vi "Conn Transaction.vi"(4 "error in (no error)":errorcluster, 5 "isolation level (chaos)":T1, 6 "operation (begin)":T3, 7 "connection reference":T2) -> (0 "error out":errorcluster, 3 "connection reference out":T2)   [LabVIEW 2017, in "NI_Database_API.lvlib"]
doc: "Begins, commits, or rolls back a transaction for any type of reference. Wire data to the reference input to determine the polymorphic instance to use or manually select the instance."
uses:
  <vilib>/addons/database/NI_Database_API.lvlib
  <vilib>/addons/database/Auxilliary.llb/DB Tools Transaction.ctl
  <vilib>/addons/database/Connection.llb/Conn ObjectReference.ctl
  <vilib>/addons/database/Auxilliary.llb/DB Tools Isolation Level.ctl
panel:
  out "ADO isolation level":i32(ring)=-1 items=["adXactUnspecified"=-1, "adXactChaos"=16, "adXactReadUncommitted, adXactBrowse"=256, "adXactCursorStability, adXactReadCommitted"=4096, "adXactRepeatableRead"=65536, "adXactSerializable, adXactIsolated"=1048576]
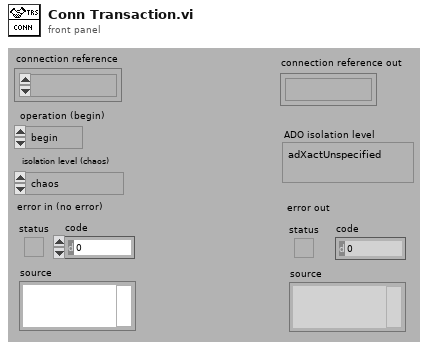
[diagram p1: front panel]
types:
  T1 = typedef "NI_Database_API.lvlib/DB Tools Isolation Level.ctl" = enum16{"chaos", "read uncommitted", "read committed", "repeatable read", "serializable"}
  T2 = typedef "NI_Database_API.lvlib/Conn ObjectReference.ctl" = refnum<k1>
  T3 = typedef "NI_Database_API.lvlib/DB Tools Transaction.ctl" = enum16{"begin", "commit", "rollback"}
  T4 = typedef "NI_Database_API.lvlib/Conn DataMembers.ctl" = cluster{"ADODB._Connection":refnum<k7>, "recordset objects":i32, "command objects":i32}
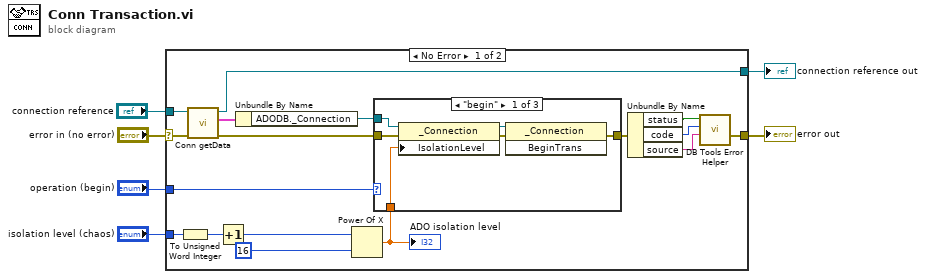
[diagram p0: block diagram]
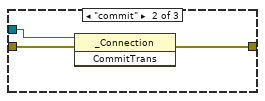
[diagram p2: hidden frame]
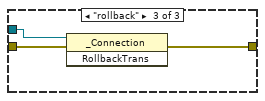
[diagram p3: hidden frame]
diagram:
  n1 = case shown="No Error" "error in (no error)" {
    selector: "error in (no error)" -> [w7 w37]
    tunnel: "operation (begin)" -> [w23 _]
    tunnel: "isolation level (chaos)" -> [w19 _]
    tunnel: "connection reference" -> [w16 w36]
    tunnel: [w14 w36] -> w3
    tunnel: [w8 w37] -> w2
    frame No Error {
      n2 = To Unsigned Word Integer(number=w19) -> (unsigned 16bit integer=w21:u16)
      n3 = call <vilib>:"Conn getData.vi"("error in (no error)"=w7, "connection reference"=w16) -> ("error out"=w15:errorcluster, "data"=w17:T4, "connection reference out"=w14:T2)  [unwired: 3 out]
      n4 = Increment(x=w21) -> (x+1=w20:u16)
      n5 = Unbundle By Name(w17) -> ("ADODB._Connection"=w13:refnum<k7>)
      n6 = Power Of X(1:u16 16 ("x"), 2:w20) -> (0:w18:dbl)
      "ADO isolation level" <- w18
      n7 = case shown="\"begin\"" w23 {
        tunnel: [w29 w32 w35] -> w9
        tunnel: w13 -> [w28 w31 w34]
        tunnel: w15 -> [w27 w30 w33]
        tunnel: w18 -> [w24 _ _]
        frame "begin" {
          n8 = property class="_Connection"(reference=w28, error in=w27, "IsolationLevel"=w24) -> (reference out=w26:refnum<k7>, error out=w25:errorcluster)
          n9 = invoke class="_Connection" method="BeginTrans"(reference=w26, error in=w25) -> (error out=w29:errorcluster)  [unwired: 1 in, 2 out]
        }
        frame "commit" {
          n10 = invoke class="_Connection" method="CommitTrans"(reference=w31, error in=w30) -> (error out=w32:errorcluster)  [unwired: 1 in, 2 out]
        }
        frame "rollback" {
          n11 = invoke class="_Connection" method="RollbackTrans"(reference=w34, error in=w33) -> (error out=w35:errorcluster)  [unwired: 1 in, 2 out]
        }
      }
      n12 = Unbundle By Name(w9) -> ("status"=w11:bool, "code"=w10:i32, "source"=w12:string)
      n13 = call <vilib>:"DB Tools Error Helper.vi"("source"=w12, "code"=w10, "status"=w11) -> ("error out"=w8:errorcluster)  [unwired: 1 in, 7 out]
    }
    frame Error {
    }
  }
  "error out" <- w2
  "connection reference out" <- w3
